vi "drawing_spline.vi"(0 "Automation Refnum in":refnum<k7>, 5 "Wpó³rzêdne X":dbl[](array[numeric]), 7 "Wspó³rzêdne Y":dbl[](array[numeric]), 9 "Wspó³rzêdne Z":dbl[](array[numeric]), 11 "error in (no error)":errorcluster) -> (15 "error out":errorcluster)   [LabVIEW 2014, in "Manipulator.lvclass"]
uses:
  Manipulator.lvclass
  <vilib>/Platform/NI_3dgraph.lvlib
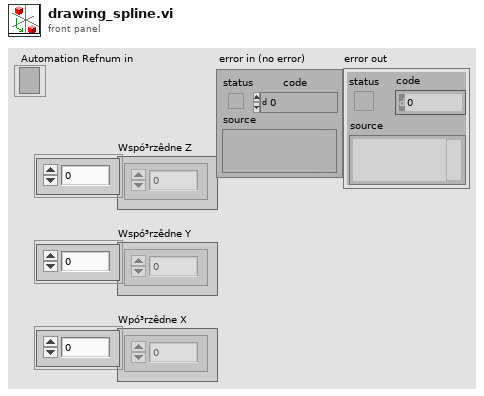
[diagram p1: front panel]
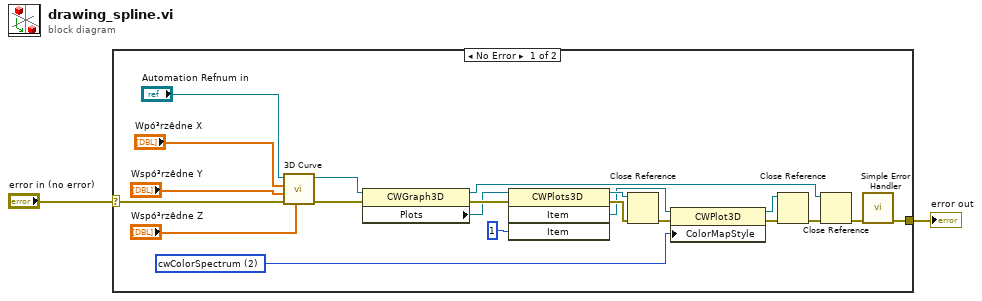
[diagram p0: block diagram]
diagram:
  n1 = case shown="No Error" "error in (no error)" {
    selector: "error in (no error)" -> [w3 w24]
    tunnel: [w4 w24] -> w2
    frame No Error {
      w7 = 2 items=["cwNone", "cwShaded", "cwColorSpectrum", "cwGrayScale"] ("ColorMapStyle")
      n2 = call <vilib>:"3D Curve.vi"("z vector"="Wspó³rzêdne Z", "error in (no error)"=w3, "y vector"="Wspó³rzêdne Y", "x vector"="Wpó³rzêdne X", "3D graph"="Automation Refnum in") -> ("error out"=w9:errorcluster, "3D graph out"=w10:refnum<k7>)  [unwired: 5 in]
      n3 = property class="CWGraph3D"(reference=w10, error in=w9) -> (reference out=w19:refnum<k7>, error out=w11:errorcluster, "Plots"=w6:refnum<k7>)
      n4 = invoke class="CWPlots3D" method="Item"(reference=w6, error in=w11, "Item"=1) -> (reference out=w13:refnum<k7>, error out=w12:errorcluster, "Item"=w8:refnum<k7>)  [unwired: 1 in, 1 out]
      n5 = Close Reference(reference=w13, error in (no error)=w12) -> (error out=w14:errorcluster)
      n6 = property class="CWPlot3D"(reference=w8, error in=w14, "ColorMapStyle"=w7) -> (reference out=w16:refnum<k7>, error out=w15:errorcluster)
      n7 = Close Reference(reference=w16, error in (no error)=w15) -> (error out=w18:errorcluster)
      n8 = Close Reference(reference=w19, error in (no error)=w18) -> (error out=w17:errorcluster)
      n9 = call <vilib>:"Simple Error Handler.vi"("error in (no error)"=w17) -> ("error out"=w4:errorcluster)  [unwired: 4 in, 4 out]
    }
    frame Error {
    }
  }
  "error out" <- w2
